vi "Dispense FN - Product Values (SubVI).vi"(1 "State Input":enum16{"OFF", "ON"}(ring), 2 "Dispense State Change?":bool, 3 "Product Weight (g)":dbl) -> (0 "Product Values":T1)   [LabVIEW 2012]
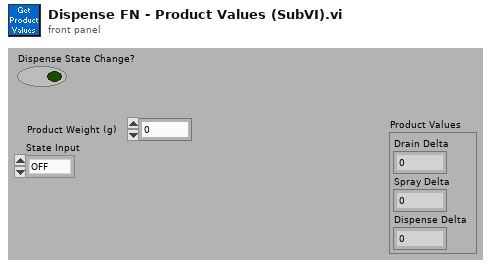
[diagram p1: front panel]
types:
  T1 = cluster{"Drain Delta":dbl, "Spray Delta":dbl, "Dispense Delta":dbl}
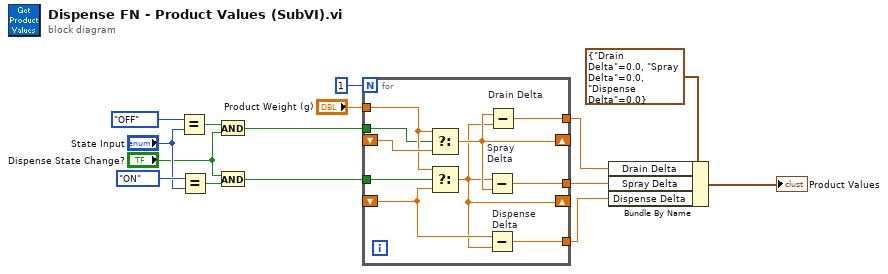
[diagram p0: block diagram]
diagram:
  n1 = Equal?(x=enum16{"OFF", "ON"}."OFF" ("Signal State 2"), y="State Input") -> (x = y?=w3:bool)
  n2 = Equal?(x=enum16{"OFF", "ON"}."ON" ("Signal State 2"), y="State Input") -> (x = y?=w7:bool)
  n3 = And(x=w3, y="Dispense State Change?") -> (x .and. y?=w1:bool)
  n4 = And(x="Dispense State Change?", y=w7) -> (x .and. y?=w6:bool)
  n5 = for {
    N: 1 -> [_]
    shift-right: [w23] -> _
    shift-left: _ -> [w25]
    shift-right: [w22] -> _
    shift-left: _ -> [w24]
    tunnel: "Product Weight (g)" -> [w21]
    tunnel: w1 -> [w20]
    tunnel: w6 -> [w19]
    tunnel: [w18] -> w12
    tunnel: [w17] -> w13
    tunnel: [w16] -> w14
    n6 = Select(t=w21, s=w20, f=w25) -> (s? t:f=w23:dbl)
    n7 = Select(t=w21, s=w19, f=w24) -> (s? t:f=w22:dbl)
    n8 = Subtract "Spray\nDelta"(x=w22, y=w23) -> (x-y=w17:dbl)
    n9 = Subtract "Dispense\nDelta"(x=w24, y=w22) -> (x-y=w16:dbl)
    n10 = Subtract "Drain Delta"(x=w23, y=w22) -> (x-y=w18:dbl)
  }
  n11 = Bundle By Name(cluster=T1 {"Drain Delta"=0.0, "Spray Delta"=0.0, "Dispense Delta"=0.0}, "Drain Delta"=w12, "Spray Delta"=w13, "Dispense Delta"=w14) -> (→"Product Values":T1)
